vi "final_control_mk9_032425.vi"() -> ()   [LabVIEW 2023]
doc: "Simplified example program for initializing the COM port, determining the data frame of up to 26 Alicats, acquiring the data of the same number of Alicats, displaying the data of the one with the selected unit ID, and writing a setpoint to the same selected unit ID.\n\nThis is a slightly more feature rich version of the Alicat Simplified Driver Example, and contains an example of a method for interfacing with up to 26 Alicats on a single COM port by means of for loops with shift registers to handle sequential commands to each included Alicat. This also contains a method to write a setpoint to the same selected unit.\n\nIf coding for multiple Alicats on a single COM port without the use of for loops with shift registers, ensure that each Alicat command is executed sequentially. Alicat's RS-232/485 does not work if multiple devices are responding simultaneously."
uses:
  <vilib>/Platform/TimedLoop/XDataNode/timing_clust.ctl
  <vilib>/Platform/TimedLoop/XDataNode/nitl_modes.ctl
  <vilib>/Platform/TimedLoop/XDataNode/wakeup.ctl
  <vilib>/DAQmx/write.llb/DAQmx Write (Analog 1D DBL NChan 1Samp).vi
  <vilib>/DAQmx/read.llb/DAQmx Read (Analog DBL 1Chan 1Samp).vi
  <extravilib>/ChannelInstances/Tag-bool/Read With Abort.vi
  <extravilib>/ChannelInstances/Tag-bool/Write With Abort.vi
  <vilib>/Utility/file.llb/Write Delimited Spreadsheet (string).vi
  <extravilib>/ChannelInstances/Tag-bool/Instantiate.vi
  <vilib>/Utility/file.llb/Read Delimited Spreadsheet (DBL).vi
  <extravilib>/ChannelInstances/Tag-bool/EndpointRead.vi
  <vilib>/DAQmx/miscellaneous.llb/DAQmx Fill In Error Info.vi
  <extravilib>/ChannelInstances/Tag-bool/Endpoint.vi
  <vilib>/platform/TimedLoop/XDataNode/XDataNode.xnode
  <vilib>/express/express arith-compare/Formula/XNode/ExpressFormulaBlockNode.xnode
  <vilib>/Platform/TimedLoop/XDataNode/XDNodeRunTimeDep.lvlib
  <extravilib>/ChannelInstances/Tag-bool.lvlib
panel:
  in  "Tab Control":enum32{"Page 1", "Page 2"}(tab)
  in  "COM Port Settings":T1={"Baud Rate"=enum."19200", "VISA Sesssion In"="MassFlowControllers"}
  out "Range Exceeded":bool
  out "Error Present":bool
  out "Error Text":string
  out "Elapsed Time [ms]\n(all units)":dbl caption="Elapsed Time (s)"
  in  "Minimum time between \nreadings [ms] (all units)":u32
  in  "Device ID's \nto Include:":T2={"A"=TRUE, "B"=TRUE, "C"=TRUE, "D"=TRUE, "E"=TRUE, "F"=TRUE, "G"=FALSE, "H"=FALSE, "I"=FALSE, "J"=FALSE, "K"=FALSE, "L"=FALSE, "M"=FALSE, "N"=FALSE, "O"=FALSE, "P"=FALSE, "Q"=FALSE, "R"=FALSE, "S"=FALSE, "T"=FALSE, "U"=FALSE, "V"=FALSE, "W"=FALSE, "X"=FALSE, "Y"=FALSE, "Z"=FALSE}
  out "Active Device":u16(ring) items=["A", "B", "C", "D", "E", "F"]
  out "Meas. Data (for active device)":T3
  in  "Write File":path
  in  "Hold Time\n[min]":dbl=17.0 min=17.0
  out "N":i32
  in  "Read File":path
  in  "End Program":bool
  in  "Start From:":i32=1
  in  "t_read [ms]":dbl=24000.0
  out "T_SCh [C]":dbl format="%0.2f"
  out "iter start":string
  out "Iter_Duration [ms]":string
  out "C_SP [ppm]":string
  out "C_H2S [ppm]":string
  in  "Start Times":path
  out "len_SP":i32
  out "Setpoints":dbl[][](array[numeric])=[[4.2, 3.3], [69.0, 4.2]]
  out "Z":dbl[](array[numeric])
  out "ASP":dbl
  out "BSP":dbl
  out "CSP":dbl
  out "DSP":dbl
  out "ESP":dbl
  out "FSP":dbl
  out "N_read":i32
  out "Iter_#":string
  out "V_D":string
  out "V_H":string
  out "all rows":dbl[][](array[numeric])
  out "T_SCh":string
  out "Iteration Duration":i64
  out "read_cnt_true":i32
  out "iter_dur_read [ms]":i64
  out "t_diff":dbl
  out "date":string
  out "time":string
  # "Totalizer Timer"
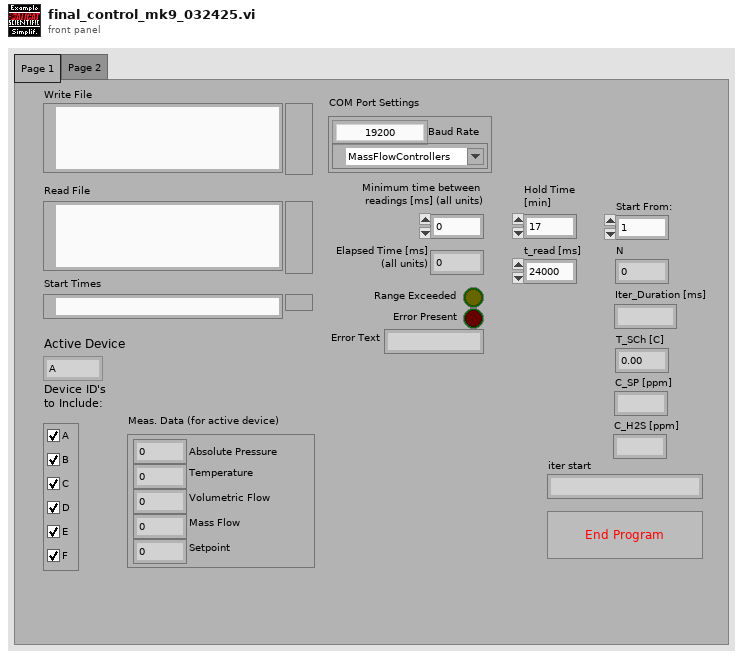
[diagram p1: front panel]
types:
  T1 = cluster{"Baud Rate":enum8{"2400", "9600", "19200", "38400", "57600", "115200", "Unknown"}, "VISA Sesssion In":refnum<visa-resource-name>}
  T2 = cluster{"A":bool, "B":bool, "C":bool, "D":bool, "E":bool, "F":bool, "G":bool, "H":bool, "I":bool, "J":bool, "K":bool, "L":bool, "M":bool, "N":bool, "O":bool, "P":bool, "Q":bool, "R":bool, "S":bool, "T":bool, "U":bool, "V":bool, "W":bool, "X":bool, "Y":bool, "Z":bool}
  T3 = cluster{"Absolute Pressure":dbl, "Gauge/Diff. Pressure":dbl, "Barometric Pressure":dbl, "Temperature":dbl, "Volumetric Flow":dbl, "Mass Flow":dbl, "Setpoint":dbl, "Valve Drive":dbl, "Totalizer":dbl, "[hr]":dbl, "[min]":dbl, "[sec]":dbl, "Totalizer Average Flow":dbl, "Totalizer Peak Flow":dbl, "Gas selected":string}
  T4 = cluster{"Unit ID":string, "Baud Rate":enum8{"2400", "9600", "19200", "38400", "57600", "115200", "Unknown"}, "VISA Sesssion In":refnum<visa-resource-name>}
  T5 = typedef "XDNodeRunTimeDep.lvlib/timing_clust.ctl" = cluster{"Expected End [f-1]":u64, "Actual End [f-1]":u64, "Finished Late? [f-1]":bool, "Expected End [i-1]":u64, "Actual End [i-1]":u64, "Finished Late? [i-1]":bool, "Expected Start [i]":u64, "Actual Start [i]":u64, "Expected Start [f]":u64, "Actual Start [f]":u64, "Source Name":string, "Structure Name":string, "Period":i64, "Deadline":i64, "Offset":i64, "Start":i64, "Priority":i32, "Timeout":i32, "Mode":T6, "Wakeup Reason":T7, "Error":errorcluster, "Source Type":string, "Secondary Source Type":string, "Global End Time":u64, "Global Start Time":u64, "Frame Duration":u64, "Iteration Duration":u64, "Assigned CPU":i32, "I/O Scan Engine Mode":u32}
  T6 = typedef "XDNodeRunTimeDep.lvlib/nitl_modes.ctl" = enum32{"No Change", "Process missed periods, maintain original phase", "Discard missed periods, maintain original phase", "Process missed periods, ignore original phase", "Discard missed periods, ignore original phase"}
  T7 = typedef "XDNodeRunTimeDep.lvlib/wakeup.ctl" = enum32{"Normal", "Aborted", "Asynchronous wakeup", "Timing source error", "Timed loop error", "Timeout"}
  T8 = typedef "Tag-bool.lvlib/))Channel.ctl" = refnum<queue>
  T9 = enum8{"2400", "9600", "19200", "38400", "57600", "115200", "Unknown"}
  T10 = cluster{"Absolute Pressure":bool, "Gauge/Diff. Pressure":bool, "Barometric Pressure":bool, "Temperature":bool, "Volumetric":bool, "Mass":bool, "Setpoint":bool, "Valve Drive":bool, "Totalizer":bool, "Totalizer Timer":bool, "Totalizer Average Flow":bool, "Totalizer Peak Flow":bool, "Gas Selected":bool, "Tot. Timer Format":u16}
  T11 = cluster{"Controller Full Scale":dbl, "Controller Select":u16, "Control Range":enum16{"Normal", "Inverted", "Bidirectional", "Unknown"}}
  T12 = cluster{"Controller Full Scale":dbl, "Controller Select":u16, "Control Range":enum16{"Normal", "Inverted", "Bidirectional", "Unknown"}}[]
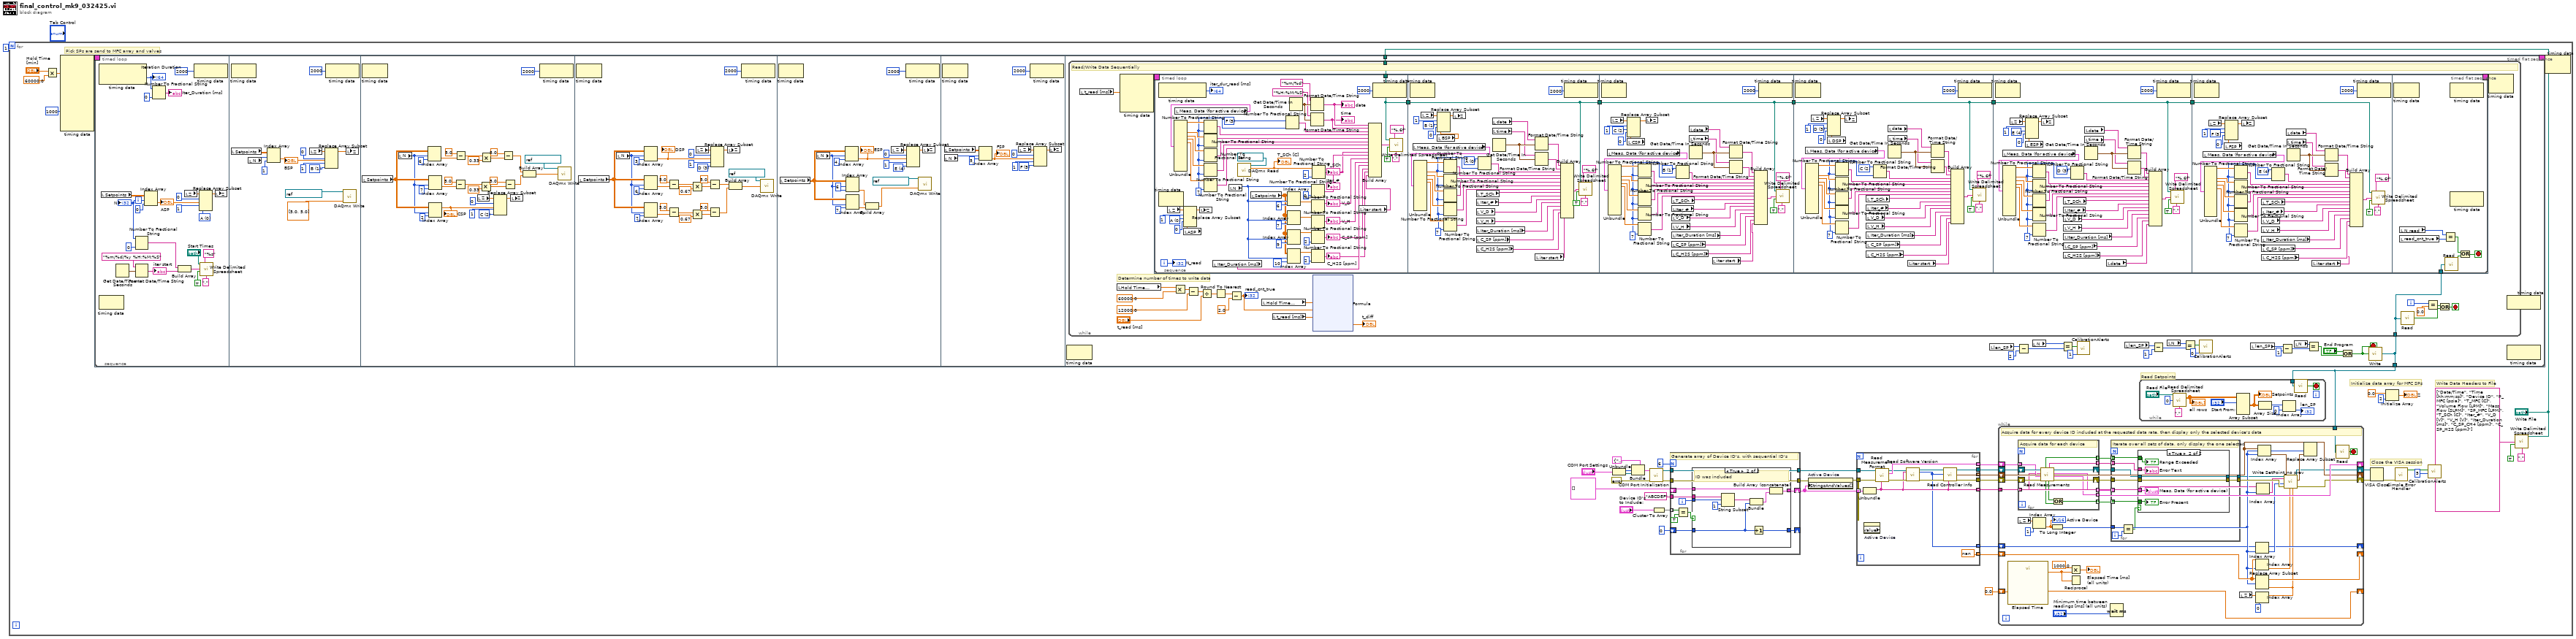
[diagram p0: block diagram]
diagram:
  n1 = for {
    N: 1 -> [_]
    # "Pick SPs are send to MFC array and valves"
    # "Write Data Headers to File"
    # "Read Setpoints"
    # "Initialize data array for MFC SPs"
    # "Close the VISA session"
    n2 = Multiply(x="Hold Time\n[min]", y=60000.0) -> (x*y=w5:dbl)
    n3 = node-c288(w5, i64 1000 ("Offset")) -> (w46:T5)  [unwired: 8 in]
    n4 = timed-loop "Write Data" {
      timing: w46 -> [_]
      timing-out: [_] -> w45
      tunnel: [w59] -> w12
      tunnel: "Write File" -> [w58]
      i -> [w67]
      stop <- w221 stop-if-true
      n5 = timed-sequence {
        timing: _ -> [_]
        timing-out: _ -> [_]
        tunnel: [w61] -> w59
        tunnel: w58 -> [w60]
        n6 = timed-flat-sequence {
          tunnel: [w216] -> w61
          tunnel: w60 -> [w217]
          frame #0 {
            w77 = u16 0 items=["A", "B", "C", "D", "E", "F"]
            n7 = node-c288() -> (w71:i64)  [unwired: 1 in, 1 out]
            "Iteration Duration" <- w71
            n8 = local read "Setpoints"() -> (w84:dbl[][])
            n9 = Get Date/Time In Seconds() -> (seconds since 1Jan1904=w72:timestamp)
            n10 = Number To Fractional String(number=w67, precision (6)=i16 0) -> (F-format string=w65:string)  [unwired: 2 in]
            n11 = Format Date/Time String(time format string (%c)="%m/%d/%y %H:%M:%S", seconds (now)=w72) -> (date/time string=w64:string)  [unwired: 1 in]
            "iter start" <- w64
            n12 = Index Array(array=w84, index (row)=w67, index (col)=0 ("index (row)")) -> (element=w82:dbl)
            "ASP" <- w82
            n13 = Number To Fractional String(number=w71, precision (6)=i16 0) -> (F-format string=→"Iter_Duration [ms]":string)  [unwired: 2 in]
            n14 = Build Array(w65, w64) -> (w63:string[])
            n15 = local read "Z"() -> (w80:dbl[])
            n16 = node-c288(i64 2000 ("Start")) -> ()  [unwired: 1 out]
            n17 = Replace Array Subset(array=w80, new element #1=w82, index #1=0 ("index"), new element #2=w77, index #2=1 ("index")) -> (w81:dbl[])
            n18 = call-poly <vilib>:"Write Delimited Spreadsheet.vi"("file path (dialog if empty)"="Start Times", "format (%s)"="%s" ("format (%.3f)"), "1D data"=w63, "append to file? (new file:F)"=TRUE, "delimiter (\\t)"="," ("delimiter (\\t)")) -> ()  [unwired: 9 in, 2 out]
            n19 = local write "Z"(w81) -> ()
            "N" <- w67
          }
          frame #1 {
            w92 = u16 1 items=["A", "B", "C", "D", "E", "F"]
            n20 = node-c288() -> ()  [unwired: 1 in, 1 out]
            n21 = local read "Setpoints"() -> (w100:dbl[][])
            n22 = local read "N"() -> (w93:i32)
            n23 = Index Array(array=w100, index (row)=w93, index (col)=1 ("index (row)")) -> (element=w97:dbl)
            "BSP" <- w97
            n24 = local read "Z"() -> (w95:dbl[])
            n25 = Replace Array Subset(array=w95, new element #1=w97, index #1=0 ("index"), new element #2=w92, index #2=1 ("index")) -> (w96:dbl[])
            n26 = node-c288(i64 2000 ("Start")) -> ()  [unwired: 1 out]
            n27 = call-poly <vilib>:"DAQmx Write.vi"("task/channels in"=refnum<k21> "Valve_cont", "data"=dbl[] [5.0, 5.0]) -> ()  [unwired: 11 in, 3 out]
            n28 = local write "Z"(w96) -> ()
          }
          frame #2 {
            w107 = u16 2 items=["A", "B", "C", "D", "E", "F"]
            n29 = node-c288() -> ()  [unwired: 1 in, 1 out]
            n30 = local read "Setpoints"() -> (w119:dbl[][])
            n31 = local read "N"() -> (w118:i32)
            n32 = Index Array(array=w119, index (row)=w118, index (col)=6 ("disabled index (col)")) -> (element=w109:dbl)
            n33 = Index Array(array=w119, index (row)=w118, index (col)=7 ("disabled index (col)")) -> (element=w117:dbl)
            n34 = Index Array(array=w119, index (row)=w118, index (col)=2 ("index (row)")) -> (element=w131:dbl)
            "CSP" <- w131
            n35 = Subtract(x=5.0, y=w117) -> (x-y=w126:dbl)
            n36 = Subtract(x=5.0, y=w109) -> (x-y=w113:dbl)
            n37 = local read "Z"() -> (w129:dbl[])
            n38 = Multiply(x=w126, y=0.33) -> (x*y=w124:dbl)
            n39 = Multiply(x=w113, y=0.33) -> (x*y=w111:dbl)
            n40 = Replace Array Subset(array=w129, new element #1=w131, index #1=0 ("index"), new element #2=w107, index #2=1 ("index")) -> (w130:dbl[])
            n41 = Subtract(x=5.0, y=w111) -> (x-y=w108:dbl)
            n42 = Subtract(x=5.0, y=w124) -> (x-y=w121:dbl)
            n43 = local write "Z"(w130) -> ()
            n44 = Build Array(w108, w121) -> (w120:dbl[])
            n45 = node-c288(i64 2000 ("Start")) -> ()  [unwired: 1 out]
            n46 = call-poly <vilib>:"DAQmx Write.vi"("task/channels in"=refnum<k21> "Valve_cont", "data"=w120) -> ()  [unwired: 11 in, 3 out]
          }
          frame #3 {
            w158 = u16 3 items=["A", "B", "C", "D", "E", "F"]
            n47 = node-c288() -> ()  [unwired: 1 in, 1 out]
            n48 = local read "Setpoints"() -> (w147:dbl[][])
            n49 = local read "N"() -> (w146:i32)
            n50 = Index Array(array=w147, index (row)=w146, index (col)=7 ("disabled index (col)")) -> (element=w139:dbl)
            n51 = Index Array(array=w147, index (row)=w146, index (col)=3 ("index (row)")) -> (element=w162:dbl)
            "DSP" <- w162
            n52 = Index Array(array=w147, index (row)=w146, index (col)=6 ("disabled index (col)")) -> (element=w145:dbl)
            n53 = Subtract(x=5.0, y=w145) -> (x-y=w155:dbl)
            n54 = Subtract(x=5.0, y=w139) -> (x-y=w143:dbl)
            n55 = Multiply(x=w155, y=0.67) -> (x*y=w153:dbl)
            n56 = Multiply(x=w143, y=0.67) -> (x*y=w141:dbl)
            n57 = local read "Z"() -> (w160:dbl[])
            n58 = Subtract(x=5.0, y=w153) -> (x-y=w149:dbl)
            n59 = Subtract(x=5.0, y=w141) -> (x-y=w138:dbl)
            n60 = Replace Array Subset(array=w160, new element #1=w162, index #1=0 ("index"), new element #2=w158, index #2=1 ("index")) -> (w161:dbl[])
            n61 = local write "Z"(w161) -> ()
            n62 = Build Array(w149, w138) -> (w148:dbl[])
            n63 = node-c288(i64 2000 ("Start")) -> ()  [unwired: 1 out]
            n64 = call-poly <vilib>:"DAQmx Write.vi"("task/channels in"=refnum<k21> "Valve_cont", "data"=w148) -> ()  [unwired: 11 in, 3 out]
          }
          frame #4 {
            w179 = u16 4 items=["A", "B", "C", "D", "E", "F"]
            n65 = node-c288() -> ()  [unwired: 1 in, 1 out]
            n66 = local read "Setpoints"() -> (w174:dbl[][])
            n67 = local read "N"() -> (w173:i32)
            n68 = Index Array(array=w174, index (row)=w173, index (col)=4 ("index (row)")) -> (element=w183:dbl)
            "ESP" <- w183
            n69 = Index Array(array=w174, index (row)=w173, index (col)=6 ("disabled index (col)")) -> (element=w176:dbl)
            n70 = Index Array(array=w174, index (row)=w173, index (col)=7 ("disabled index (col)")) -> (element=w175:dbl)
            n71 = Build Array(w176, w175) -> (w172:dbl[])
            n72 = local read "Z"() -> (w181:dbl[])
            n73 = node-c288(i64 2000 ("Start")) -> ()  [unwired: 1 out]
            n74 = Replace Array Subset(array=w181, new element #1=w183, index #1=0 ("index"), new element #2=w179, index #2=1 ("index")) -> (w182:dbl[])
            n75 = call-poly <vilib>:"DAQmx Write.vi"("task/channels in"=refnum<k21> "Valve_cont", "data"=w172) -> ()  [unwired: 11 in, 3 out]
            n76 = local write "Z"(w182) -> ()
          }
          frame #5 {
            w193 = u16 5 items=["A", "B", "C", "D", "E", "F"]
            n77 = node-c288() -> ()  [unwired: 1 in, 1 out]
            n78 = local read "Setpoints"() -> (w196:dbl[][])
            n79 = local read "N"() -> (w191:i32)
            n80 = Index Array(array=w196, index (row)=w191, index (col)=5 ("index (row)")) -> (element=w192:dbl)
            "FSP" <- w192
            n81 = local read "Z"() -> (w195:dbl[])
            n82 = node-c288(i64 2000 ("Start")) -> ()  [unwired: 1 out]
            n83 = Replace Array Subset(array=w195, new element #1=w192, index #1=0 ("index"), new element #2=w193, index #2=1 ("index")) -> (w194:dbl[])
            n84 = local write "Z"(w194) -> ()
          }
          frame #6 {
            n85 = node-c288() -> ()  [unwired: 1 in, 1 out]
            n86 = local read "len_SP"() -> (w207:i32)
            n87 = Subtract(x=w207, y=2) -> (x-y=w209:i32)
            n88 = local read "N"() -> (w208:i32)
            n89 = Equal?(x=w208, y=w209) -> (x = y?=w205:bool)
            n90 = call "CalibrationAlerts.vi"("Alert Type (0)"=1, "Trigger"=w205) -> ()  [unwired: 10 in]
            n91 = local read "len_SP"() -> (w212:i32)
            n92 = Subtract(x=w212, y=1) -> (x-y=w211:i32)
            n93 = local read "N"() -> (w215:i32)
            n94 = Equal?(x=w215, y=w211) -> (x = y?=w204:bool)
            n95 = call "CalibrationAlerts.vi"("Alert Type (0)"=0, "Trigger"=w204) -> ()  [unwired: 10 in]
            n96 = local read "len_SP"() -> (w220:i32)
            n97 = Subtract(x=w220, y=1) -> (x-y=w223:i32)
            n98 = local read "N"() -> (w219:i32)
            n99 = Equal?(x=w219, y=w223) -> (x = y?=w222:bool)
            n100 = Or(x="End Program", y=w222) -> (x .or. y?=w221:bool)
            n101 = call <extravilib>:"Write.vi"("element"=w221) -> ("channel"=w216:T8)  [unwired: 1 out]
            n102 = while {
              tunnel: w217 -> [w245]
              tunnel: w216 -> [w235]
              i -> [w234]
              stop <- w241 stop-if-true
              # "Determine number of times to write data"
              # "Read/Write Data Sequentially"
              n103 = local read "t_read [ms]"() -> (w225:dbl)
              n104 = local read "Hold Time\n[min]"() -> (w239:dbl)
              n105 = node-c288(w225) -> (w247:T5)  [unwired: 3 in]
              n106 = timed-loop {
                timing: w247 -> [_]
                timing-out: [_] -> w246
                tunnel: w245 -> [w260]
                tunnel: w235 -> [w261]
                i -> [w325]
                stop <- w549 stop-if-true
                n107 = timed-sequence {
                  timing: _ -> [_]
                  timing-out: _ -> [_]
                  tunnel: w261 -> [w263]
                  tunnel: w260 -> [w262]
                  n108 = timed-flat-sequence {
                    tunnel: [w291] -> w268
                    tunnel: w262 -> [w291]
                    tunnel: w268 -> [w357]
                    tunnel: [w357] -> w267
                    tunnel: w267 -> [w393]
                    tunnel: [w393] -> w266
                    tunnel: w266 -> [w432]
                    tunnel: [w432] -> w265
                    tunnel: w265 -> [w465]
                    tunnel: [w465] -> w264
                    tunnel: w264 -> [w518]
                    tunnel: w263 -> [w548]
                    frame #0 {
                      w306 = u16 5 items=["A", "B", "C", "D", "E", "F"]
                      w309 = u16 0 items=["A", "B", "C", "D", "E", "F"]
                      w302 = i16 7 ("precision (6)")
                      n109 = node-c288() -> (→"iter_dur_read [ms]":i64)  [unwired: 1 in]
                      n110 = local read "Z"() -> (w295:dbl[])
                      n111 = local read "Meas. Data (for active device)"() -> (w292:T3)
                      n112 = Unbundle(w292) -> ("Absolute Pressure"=w315:dbl, "Temperature"=w305:dbl, "Volumetric Flow"=w311:dbl, "Mass Flow"=w304:dbl, "Setpoint"=w303:dbl)  [unwired: 10 out]
                      n113 = local read "ASP"() -> (w293:dbl)
                      n114 = Replace Array Subset(array=w295, new element #1=w309, index #1=1 ("index"), new element #2=w293, index #2=0 ("index")) -> (w294:dbl[])
                      n115 = local write "Z"(w294) -> ()
                      n116 = Number To Fractional String(number=w315, precision (6)=w302) -> (F-format string=w300:string)  [unwired: 2 in]
                      n117 = Number To Fractional String(number=w305, precision (6)=w302) -> (F-format string=w298:string)  [unwired: 2 in]
                      n118 = Number To Fractional String(number=w311, precision (6)=w302) -> (F-format string=w299:string)  [unwired: 2 in]
                      n119 = Number To Fractional String(number=w304, precision (6)=w302) -> (F-format string=w297:string)  [unwired: 2 in]
                      n120 = Number To Fractional String(number=w303, precision (6)=w302) -> (F-format string=w296:string)  [unwired: 2 in]
                      n121 = local read "Iter_Duration [ms]"() -> (w290:string)
                      n122 = local read "N"() -> (w272:i32)
                      n123 = call-poly <vilib>:"DAQmx Read.vi"("task/channels in"=refnum<k21> "T_SCh") -> ("data"=w318:dbl)  [unwired: 12 in, 2 out]
                      "T_SCh [C]" <- w318
                      n124 = local read "Setpoints"() -> (w271:dbl[][])
                      n125 = Number To Fractional String(number=w306, precision (6)=w302) -> (F-format string=w301:string)  [unwired: 2 in]
                      n126 = Index Array(array=w271, index (row)=w272, index (col)=6 ("disabled index (col)")) -> (element=w322:dbl)
                      n127 = Index Array(array=w271, index (row)=w272, index (col)=7 ("disabled index (col)")) -> (element=w321:dbl)
                      n128 = Index Array(array=w271, index (row)=w272, index (col)=9 ("disabled index (col)")) -> (element=w278:dbl)
                      n129 = Index Array(array=w271, index (row)=w272, index (col)=10 ("disabled index (col)")) -> (element=w274:dbl)
                      n130 = Get Date/Time In Seconds() -> (seconds since 1Jan1904=w284:timestamp)
                      n131 = Format Date/Time String(time format string (%c)="%m/%d", seconds (now)=w284) -> (date/time string=w286:string)  [unwired: 1 in]
                      "date" <- w286
                      n132 = Format Date/Time String(time format string (%c)="%H:%M:%S", seconds (now)=w284) -> (date/time string=w285:string)  [unwired: 1 in]
                      "time" <- w285
                      n133 = Number To Fractional String(number=w272, precision (6)=i16 0) -> (F-format string=w287:string)  [unwired: 2 in]
                      "Iter_#" <- w287
                      n134 = Number To Fractional String(number=w322) -> (F-format string=w288:string)  [unwired: 3 in]
                      "V_D" <- w288
                      n135 = Number To Fractional String(number=w321) -> (F-format string=w289:string)  [unwired: 3 in]
                      "V_H" <- w289
                      n136 = Number To Fractional String(number=w278, precision (6)=i16 2) -> (F-format string=w276:string)  [unwired: 2 in]
                      "C_SP [ppm]" <- w276
                      n137 = Number To Fractional String(number=w274, precision (6)=i16 2) -> (F-format string=w270:string)  [unwired: 2 in]
                      "C_H2S [ppm]" <- w270
                      n138 = Number To Fractional String(number=w318, precision (6)=i16 2) -> (F-format string=w281:string)  [unwired: 2 in]
                      "T_SCh" <- w281
                      n139 = local read "iter start"() -> (w269:string)
                      n140 = Build Array(w286, w285, w301, w300, w298, w299, w297, w296, w281, w287, w288, w289, w290, w276, w270, w269) -> (w312:string[])
                      n141 = node-c288(i64 2000 ("Start")) -> ()  [unwired: 1 out]
                      n142 = call-poly <vilib>:"Write Delimited Spreadsheet.vi"("file path (dialog if empty)"=w291, "format (%s)"="%.6f" ("format (%.3f)"), "1D data"=w312, "append to file? (new file:F)"=TRUE, "delimiter (\\t)"="," ("delimiter (\\t)")) -> ()  [unwired: 9 in, 2 out]
                      "N_read" <- w325
                    }
                    frame #1 {
                      w354 = u16 0 items=["A", "B", "C", "D", "E", "F"]
                      w363 = u16 1 items=["A", "B", "C", "D", "E", "F"]
                      w350 = i16 7 ("precision (6)")
                      n143 = node-c288() -> ()  [unwired: 1 in, 1 out]
                      n144 = local read "Meas. Data (for active device)"() -> (w361:T3)
                      n145 = Unbundle(w361) -> ("Absolute Pressure"=w369:dbl, "Temperature"=w353:dbl, "Volumetric Flow"=w365:dbl, "Mass Flow"=w352:dbl, "Setpoint"=w351:dbl)  [unwired: 10 out]
                      n146 = local read "Z"() -> (w360:dbl[])
                      n147 = local read "BSP"() -> (w355:dbl)
                      n148 = Replace Array Subset(array=w360, new element #1=w363, index #1=1 ("index"), new element #2=w355, index #2=0 ("index")) -> (w359:dbl[])
                      n149 = Number To Fractional String(number=w369, precision (6)=w350) -> (F-format string=w348:string)  [unwired: 2 in]
                      n150 = Number To Fractional String(number=w353, precision (6)=w350) -> (F-format string=w346:string)  [unwired: 2 in]
                      n151 = Number To Fractional String(number=w365, precision (6)=w350) -> (F-format string=w347:string)  [unwired: 2 in]
                      n152 = Number To Fractional String(number=w352, precision (6)=w350) -> (F-format string=w345:string)  [unwired: 2 in]
                      n153 = Number To Fractional String(number=w351, precision (6)=w350) -> (F-format string=w344:string)  [unwired: 2 in]
                      n154 = local write "Z"(w359) -> ()
                      n155 = local read "T_SCh"() -> (w343:string)
                      n156 = local read "Iter_#"() -> (w342:string)
                      n157 = local read "V_D"() -> (w341:string)
                      n158 = local read "V_H"() -> (w340:string)
                      n159 = local read "Iter_Duration [ms]"() -> (w339:string)
                      n160 = local read "C_SP [ppm]"() -> (w333:string)
                      n161 = local read "C_H2S [ppm]"() -> (w332:string)
                      n162 = Number To Fractional String(number=w354, precision (6)=w350) -> (F-format string=w349:string)  [unwired: 2 in]
                      n163 = local read "date"() -> (w334:string)
                      n164 = local read "time"() -> (w335:string)
                      n165 = Get Date/Time In Seconds() -> (seconds since 1Jan1904=w336:timestamp)
                      n166 = Format Date/Time String(time format string (%c)=w334, seconds (now)=w336) -> (date/time string=w338:string)  [unwired: 1 in]
                      n167 = Format Date/Time String(time format string (%c)=w335, seconds (now)=w336) -> (date/time string=w337:string)  [unwired: 1 in]
                      n168 = local read "iter start"() -> (w331:string)
                      n169 = Build Array(w338, w337, w349, w348, w346, w347, w345, w344, w343, w342, w341, w340, w339, w333, w332, w331) -> (w366:string[])
                      n170 = node-c288(i64 2000 ("Start")) -> ()  [unwired: 1 out]
                      n171 = call-poly <vilib>:"Write Delimited Spreadsheet.vi"("file path (dialog if empty)"=w357, "format (%s)"="%.6f" ("format (%.3f)"), "1D data"=w366, "append to file? (new file:F)"=TRUE, "delimiter (\\t)"="," ("delimiter (\\t)")) -> ()  [unwired: 9 in, 2 out]
                    }
                    frame #2 {
                      w399 = u16 1 items=["A", "B", "C", "D", "E", "F"]
                      w398 = i16 7 ("precision (6)")
                      w411 = u16 2 items=["A", "B", "C", "D", "E", "F"]
                      n172 = node-c288() -> ()  [unwired: 1 in, 1 out]
                      n173 = local read "Meas. Data (for active device)"() -> (w400:T3)
                      n174 = Unbundle(w400) -> ("Absolute Pressure"=w405:dbl, "Temperature"=w403:dbl, "Volumetric Flow"=w404:dbl, "Mass Flow"=w402:dbl, "Setpoint"=w401:dbl)  [unwired: 10 out]
                      n175 = local read "Z"() -> (w410:dbl[])
                      n176 = local read "CSP"() -> (w406:dbl)
                      n177 = Replace Array Subset(array=w410, new element #1=w411, index #1=1 ("index"), new element #2=w406, index #2=0 ("index")) -> (w409:dbl[])
                      n178 = Number To Fractional String(number=w405, precision (6)=w398) -> (F-format string=w386:string)  [unwired: 2 in]
                      n179 = Number To Fractional String(number=w403, precision (6)=w398) -> (F-format string=w385:string)  [unwired: 2 in]
                      n180 = Number To Fractional String(number=w404, precision (6)=w398) -> (F-format string=w384:string)  [unwired: 2 in]
                      n181 = Number To Fractional String(number=w402, precision (6)=w398) -> (F-format string=w383:string)  [unwired: 2 in]
                      n182 = Number To Fractional String(number=w401, precision (6)=w398) -> (F-format string=w382:string)  [unwired: 2 in]
                      n183 = local write "Z"(w409) -> ()
                      n184 = local read "T_SCh"() -> (w392:string)
                      n185 = local read "Iter_#"() -> (w391:string)
                      n186 = local read "V_D"() -> (w390:string)
                      n187 = local read "V_H"() -> (w389:string)
                      n188 = local read "Iter_Duration [ms]"() -> (w388:string)
                      n189 = local read "C_SP [ppm]"() -> (w376:string)
                      n190 = local read "C_H2S [ppm]"() -> (w375:string)
                      n191 = Number To Fractional String(number=w399, precision (6)=w398) -> (F-format string=w387:string)  [unwired: 2 in]
                      n192 = local read "date"() -> (w377:string)
                      n193 = local read "time"() -> (w378:string)
                      n194 = Get Date/Time In Seconds() -> (seconds since 1Jan1904=w379:timestamp)
                      n195 = local read "iter start"() -> (w374:string)
                      n196 = Format Date/Time String(time format string (%c)=w377, seconds (now)=w379) -> (date/time string=w381:string)  [unwired: 1 in]
                      n197 = Format Date/Time String(time format string (%c)=w378, seconds (now)=w379) -> (date/time string=w380:string)  [unwired: 1 in]
                      n198 = Build Array(w381, w380, w387, w386, w385, w384, w383, w382, w392, w391, w390, w389, w388, w376, w375, w374) -> (w394:string[])
                      n199 = node-c288(i64 2000 ("Start")) -> ()  [unwired: 1 out]
                      n200 = call-poly <vilib>:"Write Delimited Spreadsheet.vi"("file path (dialog if empty)"=w393, "format (%s)"="%.6f" ("format (%.3f)"), "1D data"=w394, "append to file? (new file:F)"=TRUE, "delimiter (\\t)"="," ("delimiter (\\t)")) -> ()  [unwired: 9 in, 2 out]
                    }
                    frame #3 {
                      w426 = u16 3 items=["A", "B", "C", "D", "E", "F"]
                      w449 = u16 2 items=["A", "B", "C", "D", "E", "F"]
                      w448 = i16 7 ("precision (6)")
                      n201 = node-c288() -> ()  [unwired: 1 in, 1 out]
                      n202 = local read "Meas. Data (for active device)"() -> (w431:T3)
                      n203 = Unbundle(w431) -> ("Absolute Pressure"=w454:dbl, "Temperature"=w452:dbl, "Volumetric Flow"=w453:dbl, "Mass Flow"=w451:dbl, "Setpoint"=w450:dbl)  [unwired: 10 out]
                      n204 = local read "Z"() -> (w429:dbl[])
                      n205 = local read "DSP"() -> (w430:dbl)
                      n206 = Replace Array Subset(array=w429, new element #1=w426, index #1=1 ("index"), new element #2=w430, index #2=0 ("index")) -> (w428:dbl[])
                      n207 = Number To Fractional String(number=w454, precision (6)=w448) -> (F-format string=w442:string)  [unwired: 2 in]
                      n208 = Number To Fractional String(number=w452, precision (6)=w448) -> (F-format string=w441:string)  [unwired: 2 in]
                      n209 = Number To Fractional String(number=w453, precision (6)=w448) -> (F-format string=w440:string)  [unwired: 2 in]
                      n210 = Number To Fractional String(number=w451, precision (6)=w448) -> (F-format string=w439:string)  [unwired: 2 in]
                      n211 = Number To Fractional String(number=w450, precision (6)=w448) -> (F-format string=w438:string)  [unwired: 2 in]
                      n212 = local write "Z"(w428) -> ()
                      n213 = local read "T_SCh"() -> (w433:string)
                      n214 = local read "Iter_#"() -> (w434:string)
                      n215 = local read "V_D"() -> (w435:string)
                      n216 = local read "V_H"() -> (w436:string)
                      n217 = local read "Iter_Duration [ms]"() -> (w437:string)
                      n218 = local read "C_SP [ppm]"() -> (w419:string)
                      n219 = local read "C_H2S [ppm]"() -> (w418:string)
                      n220 = Number To Fractional String(number=w449, precision (6)=w448) -> (F-format string=w443:string)  [unwired: 2 in]
                      n221 = local read "date"() -> (w420:string)
                      n222 = local read "time"() -> (w421:string)
                      n223 = Get Date/Time In Seconds() -> (seconds since 1Jan1904=w422:timestamp)
                      n224 = local read "iter start"() -> (w417:string)
                      n225 = Format Date/Time String(time format string (%c)=w420, seconds (now)=w422) -> (date/time string=w424:string)  [unwired: 1 in]
                      n226 = Format Date/Time String(time format string (%c)=w421, seconds (now)=w422) -> (date/time string=w423:string)  [unwired: 1 in]
                      n227 = Build Array(w424, w423, w443, w442, w441, w440, w439, w438, w433, w434, w435, w436, w437, w419, w418, w417) -> (w444:string[])
                      n228 = node-c288(i64 2000 ("Start")) -> ()  [unwired: 1 out]
                      n229 = call-poly <vilib>:"Write Delimited Spreadsheet.vi"("file path (dialog if empty)"=w432, "format (%s)"="%.6f" ("format (%.3f)"), "1D data"=w444, "append to file? (new file:F)"=TRUE, "delimiter (\\t)"="," ("delimiter (\\t)")) -> ()  [unwired: 9 in, 2 out]
                    }
                    frame #4 {
                      w473 = u16 4 items=["A", "B", "C", "D", "E", "F"]
                      w492 = u16 3 items=["A", "B", "C", "D", "E", "F"]
                      w491 = i16 7 ("precision (6)")
                      n230 = node-c288() -> ()  [unwired: 1 in, 1 out]
                      n231 = local read "Meas. Data (for active device)"() -> (w475:T3)
                      n232 = Unbundle(w475) -> ("Absolute Pressure"=w497:dbl, "Temperature"=w495:dbl, "Volumetric Flow"=w496:dbl, "Mass Flow"=w494:dbl, "Setpoint"=w493:dbl)  [unwired: 10 out]
                      n233 = local read "Z"() -> (w470:dbl[])
                      n234 = local read "ESP"() -> (w471:dbl)
                      n235 = Replace Array Subset(array=w470, new element #1=w473, index #1=1 ("index"), new element #2=w471, index #2=0 ("index")) -> (w469:dbl[])
                      n236 = Number To Fractional String(number=w497, precision (6)=w491) -> (F-format string=w485:string)  [unwired: 2 in]
                      n237 = Number To Fractional String(number=w495, precision (6)=w491) -> (F-format string=w484:string)  [unwired: 2 in]
                      n238 = Number To Fractional String(number=w496, precision (6)=w491) -> (F-format string=w483:string)  [unwired: 2 in]
                      n239 = Number To Fractional String(number=w494, precision (6)=w491) -> (F-format string=w482:string)  [unwired: 2 in]
                      n240 = Number To Fractional String(number=w493, precision (6)=w491) -> (F-format string=w481:string)  [unwired: 2 in]
                      n241 = local write "Z"(w469) -> ()
                      n242 = local read "T_SCh"() -> (w480:string)
                      n243 = local read "Iter_#"() -> (w476:string)
                      n244 = local read "V_D"() -> (w477:string)
                      n245 = local read "V_H"() -> (w478:string)
                      n246 = local read "Iter_Duration [ms]"() -> (w479:string)
                      n247 = local read "C_SP [ppm]"() -> (w462:string)
                      n248 = local read "C_H2S [ppm]"() -> (w461:string)
                      n249 = Number To Fractional String(number=w492, precision (6)=w491) -> (F-format string=w486:string)  [unwired: 2 in]
                      n250 = local read "date"() -> (w463:string)
                      n251 = local read "time"() -> (w464:string)
                      n252 = Get Date/Time In Seconds() -> (seconds since 1Jan1904=w466:timestamp)
                      n253 = local read "date"() -> (w460:string)
                      n254 = Format Date/Time String(time format string (%c)=w463, seconds (now)=w466) -> (date/time string=w468:string)  [unwired: 1 in]
                      n255 = Format Date/Time String(time format string (%c)=w464, seconds (now)=w466) -> (date/time string=w467:string)  [unwired: 1 in]
                      n256 = Build Array(w468, w467, w486, w485, w484, w483, w482, w481, w480, w476, w477, w478, w479, w462, w461, w460) -> (w487:string[])
                      n257 = node-c288(i64 2000 ("Start")) -> ()  [unwired: 1 out]
                      n258 = call-poly <vilib>:"Write Delimited Spreadsheet.vi"("file path (dialog if empty)"=w465, "format (%s)"="%.6f" ("format (%.3f)"), "1D data"=w487, "append to file? (new file:F)"=TRUE, "delimiter (\\t)"="," ("delimiter (\\t)")) -> ()  [unwired: 9 in, 2 out]
                    }
                    frame #5 {
                      w516 = u16 5 items=["A", "B", "C", "D", "E", "F"]
                      w536 = u16 4 items=["A", "B", "C", "D", "E", "F"]
                      w535 = i16 7 ("precision (6)")
                      n259 = node-c288() -> ()  [unwired: 1 in, 1 out]
                      n260 = local read "Meas. Data (for active device)"() -> (w519:T3)
                      n261 = Unbundle(w519) -> ("Absolute Pressure"=w541:dbl, "Temperature"=w539:dbl, "Volumetric Flow"=w540:dbl, "Mass Flow"=w538:dbl, "Setpoint"=w537:dbl)  [unwired: 10 out]
                      n262 = local read "Z"() -> (w512:dbl[])
                      n263 = local read "FSP"() -> (w514:dbl)
                      n264 = Replace Array Subset(array=w512, new element #1=w516, index #1=1 ("index"), new element #2=w514, index #2=0 ("index")) -> (w513:dbl[])
                      n265 = Number To Fractional String(number=w541, precision (6)=w535) -> (F-format string=w529:string)  [unwired: 2 in]
                      n266 = Number To Fractional String(number=w539, precision (6)=w535) -> (F-format string=w528:string)  [unwired: 2 in]
                      n267 = Number To Fractional String(number=w540, precision (6)=w535) -> (F-format string=w527:string)  [unwired: 2 in]
                      n268 = Number To Fractional String(number=w538, precision (6)=w535) -> (F-format string=w526:string)  [unwired: 2 in]
                      n269 = Number To Fractional String(number=w537, precision (6)=w535) -> (F-format string=w525:string)  [unwired: 2 in]
                      n270 = local write "Z"(w513) -> ()
                      n271 = local read "T_SCh"() -> (w520:string)
                      n272 = local read "Iter_#"() -> (w521:string)
                      n273 = local read "V_D"() -> (w522:string)
                      n274 = local read "V_H"() -> (w523:string)
                      n275 = local read "Iter_Duration [ms]"() -> (w524:string)
                      n276 = local read "C_SP [ppm]"() -> (w506:string)
                      n277 = local read "C_H2S [ppm]"() -> (w505:string)
                      n278 = Number To Fractional String(number=w536, precision (6)=w535) -> (F-format string=w530:string)  [unwired: 2 in]
                      n279 = local read "date"() -> (w507:string)
                      n280 = local read "time"() -> (w508:string)
                      n281 = Get Date/Time In Seconds() -> (seconds since 1Jan1904=w509:timestamp)
                      n282 = local read "iter start"() -> (w504:string)
                      n283 = Format Date/Time String(time format string (%c)=w507, seconds (now)=w509) -> (date/time string=w511:string)  [unwired: 1 in]
                      n284 = Format Date/Time String(time format string (%c)=w508, seconds (now)=w509) -> (date/time string=w510:string)  [unwired: 1 in]
                      n285 = Build Array(w511, w510, w530, w529, w528, w527, w526, w525, w520, w521, w522, w523, w524, w506, w505, w504) -> (w531:string[])
                      n286 = node-c288(i64 2000 ("Start")) -> ()  [unwired: 1 out]
                      n287 = call-poly <vilib>:"Write Delimited Spreadsheet.vi"("file path (dialog if empty)"=w518, "format (%s)"="%.6f" ("format (%.3f)"), "1D data"=w531, "append to file? (new file:F)"=TRUE, "delimiter (\\t)"="," ("delimiter (\\t)")) -> ()  [unwired: 9 in, 2 out]
                    }
                    frame #6 {
                      n288 = node-c288() -> ()  [unwired: 1 in, 1 out]
                      n289 = local read "N_read"() -> (w546:i32)
                      n290 = local read "read_cnt_true"() -> (w547:i32)
                      n291 = Equal?(x=w546, y=w547) -> (x = y?=w551:bool)
                      n292 = call <extravilib>:"Read.vi"("channel"=w548) -> ("element"=w550:bool)  [unwired: 1 in, 1 out]
                      n293 = node-c288() -> ()  [unwired: 1 in, 1 out]
                      n294 = Or(x=w551, y=w550) -> (x .or. y?=w549:bool)
                    }
                  }
                }
                n295 = node-c288() -> ()  [unwired: 1 in, 1 out]
                n296 = node-c288() -> ()  [unwired: 1 in, 1 out]
              }
              n297 = Multiply(x=w239, y=60000.0) -> (x*y=w238:dbl)
              n298 = Subtract(x=w238, y=12000.0) -> (x-y=w236:dbl)
              n299 = Divide(x=w236, y="t_read [ms]") -> (x/y=w232:dbl)
              n300 = Round To Nearest(number=w232) -> (nearest integer value=w231:dbl)
              n301 = Subtract(x=w231, y=2.0) -> (x-y=w226:dbl)
              "read_cnt_true" <- w226
              n302 = local read "Hold Time\n[min]"() -> (w228:dbl)
              n303 = local read "t_read [ms]"() -> (w227:dbl)
              n304 = xnode "Formula"("X1"=w228, "X2"=w226, "X3"=w227) -> ("Result"=→"t_diff":dbl)  [unwired: 1 in, 1 out]
              n305 = call <extravilib>:"Read.vi"("channel"=w235) -> ("element"=w242:bool)  [unwired: 1 in, 1 out]
              n306 = Equal?(x=w234, y=0.0) -> (x = y?=w243:bool)
              n307 = Or(x=w243, y=w242) -> (x .or. y?=w241:bool)
              n308 = node-c288(w246) -> ()  [unwired: 1 out]
            }
            n309 = node-c288() -> ()  [unwired: 1 in, 1 out]
          }
        }
      }
      n310 = node-c288() -> ()  [unwired: 1 in, 1 out]
      n311 = node-c288() -> ()  [unwired: 1 in, 1 out]
    }
    n312 = Unbundle("COM Port Settings") -> ("Baud Rate"=w37:T9, "VISA Sesssion In"=w36:refnum<visa-resource-name>)
    n313 = Bundle(cluster=T4 {"Unit ID"="A", "Baud Rate"=enum."19200", "VISA Sesssion In"="COM1"} ("Communication Settings"), "Baud Rate"=w37, "VISA Sesssion In"=w36) -> (w35:T4)  [unwired: 1 in]
    n314 = call "COM Port Initialization.vi"("error in (no error)"=errorcluster {"status"=FALSE, "code"=0, "source"=""}, "Communication Settings"=w35) -> ("error out"=w28:errorcluster, "VISA Session Out"=w27:refnum<visa-resource-name>)  [unwired: 8 in]
    n315 = Cluster To Array(cluster="Device ID's \nto Include:") -> (array=w31:bool[])
    n316 = for {
      N: 6 -> [_]
      tunnel: "ABCDEF" -> [w593]
      tunnel: w31 -> [w586] mode=indexing
      shift-right: [w585] -> _
      shift-left: u16 0 ("length (rest)") -> [w591]
      shift-right: [w590] -> w25
      shift-left: cluster{string, u16}[] [] -> [w589]
      tunnel: w28 -> [w584]
      tunnel: w27 -> [w583]
      tunnel: [w584] -> w18
      tunnel: [w583] -> w26
      i -> [w592]
      # "Generate array of Device ID's, with sequential ID's"
      n317 = Equal?(x=w586, y=TRUE) -> (x = y?=w588:bool)
      n318 = case shown="True" w588 {
        tunnel: w593 -> [_ w604]
        tunnel: w592 -> [_ w603]
        tunnel: w591 -> [w594 w596]
        tunnel: [w595 w599] -> w590
        tunnel: w589 -> [w595 w597]
        tunnel: [w594 w600] -> w585
        frame False {
          # "ID was not included"
        }
        frame True {
          # "ID was included"
          n319 = String Subset(string=w604, offset (0)=w603, length (rest)=1 ("length (rest)")) -> (substring=w601:string)
          n320 = Bundle(w601, "length (rest)"=w596) -> (w598:cluster{string, "length (rest)":u16})  [unwired: 1 in]
          n321 = Increment(x=w596) -> (x+1=w600:u16)
          n322 = Build Array (concatenate)(w597, w598) -> (w599:cluster{string, "length (rest)":u16}[])
        }
      }
    }
    n323 = property on="Active Device" class="Ring (strict)"(error in=w18, "StringsAndValues[]"=w25) -> (error out=w17:errorcluster)  [unwired: 1 in, 1 out]
    n324 = for {
      tunnel: w26 -> [w581]
      tunnel: [w578] -> w22
      tunnel: w17 -> [w582]
      tunnel: [w577] -> w21
      tunnel: w25 -> [w579] mode=indexing
      tunnel: [w580] -> w24 mode=indexing
      tunnel: [w570] -> w23 mode=indexing
      tunnel: [w576] -> w20 mode=indexing
      tunnel: [nan ("Setpoint")] -> w19 mode=indexing
      tunnel: [w569] -> w16 mode=indexing
      # "Get measurement formats, unit ID's and the controller info"
      n325 = Unbundle(w579) -> (w570:string)  [unwired: 1 out]
      n326 = property on="Active Device" class="Ring (strict)" props=["Value"]() -> ()  [unwired: 2 in, 3 out]
      n327 = call "Read Measurement Format.vi"("Unit ID (A)"=w570, "error in"=w582, "VISA Session In"=w581) -> ("error out"=w573:errorcluster, "Data Frame Format"=w580:T10, "VISA Session Out"=w574:refnum<visa-resource-name>)  [unwired: 6 in]
      n328 = call "Read Software Version.vi"("Unit ID (A)"=w570, "error in"=w573, "VISA Session In"=w574) -> ("error out"=w572:errorcluster, "Software Version"=w569:u8, "VISA Session Out"=w571:refnum<visa-resource-name>)  [unwired: 6 in]
      n329 = call "Read Controller Info.vi"("Unit ID (A)"=w570, "error in"=w572, "Software Version"=w569, "VISA Session In"=w571) -> ("error out"=w577:errorcluster, "Controller Info out"=w576:T11, "VISA Session Out"=w578:refnum<visa-resource-name>)  [unwired: 4 in, 1 out]
    }
    n330 = while {
      shift-right: [w641] -> _
      shift-left: 0.0 ("Set Start Time (s)") -> [w644]
      shift-right: [w627] -> w40
      shift-left: w21 -> [w643]
      shift-right: [w608] -> w41
      shift-left: w22 -> [w642]
      tunnel: w23 -> [w606]
      shift-right: [w629] -> _
      shift-left: w24 -> [w636]
      shift-right: [w626] -> _
      shift-left: w20 -> [w624]
      shift-right: [w622] -> _
      shift-left: w19 -> [w621]
      shift-right: [w617] -> _
      shift-left: w16 -> [w617]
      tunnel: w12 -> [w615]
      stop <- w616 stop-if-true
      # "Acquire data for every device ID included at the requested data rate, then display only the selected device's data"
      n331 = call "Elapsed Time"("Set Start Time (s)"=w644) -> ("Get Start Time (s)"=w641:dbl, "Elapsed Time (s)"=w638:dbl)  [unwired: 11 in, 6 out]
      n332 = for {
        shift-right: [w673] -> w635
        shift-left: w643 -> [w676]
        shift-right: [w674] -> w634
        shift-left: w642 -> [w675]
        tunnel: w636 -> [w670] mode=indexing
        tunnel: w606 -> [w669] mode=indexing
        tunnel: [w668] -> w633 mode=indexing
        tunnel: [w667] -> w632 mode=indexing
        tunnel: [w666] -> w631 mode=indexing
        tunnel: [w665] -> w630 mode=indexing
        tunnel: [w664] -> w629 mode=indexing
        # "Acquire data for each device"
        n333 = call "Read Measurements.vi"("error in"=w676, "Data Frame Format In"=w670, "Unit ID (A)"=w669, "VISA Session In"=w675) -> ("error out"=w673:errorcluster, "Data Frame Format Out"=w664:T10, "Data Cluster"=w667:T3, "VISA Session Out"=w674:refnum<visa-resource-name>, "Unknown Dataframe Info"=w672:bool, "Error/Overrange/Unknown String"=w666:string, "Error Present"=w671:bool, "Range Exceeded"=w665:bool)
        n334 = Or(x=w672, y=w671) -> (x .or. y?=w668:bool)
      }
      n335 = local read "Z"() -> (w612:dbl[])
      n336 = Index Array(array=w612, index=1 ("index (row)")) -> (element=w610:dbl)
      "Active Device" <- w610
      n337 = To Long Integer(number=w610) -> (32bit integer=w619:i32)
      n338 = Multiply(x=1000.0 ("y"), y=w638) -> (x*y=→"Elapsed Time [ms]\n(all units)":dbl)
      n339 = Reciprocal(x=w638) -> ()  [unwired: 1 out]
      n340 = Wait (ms)(milliseconds to wait="Minimum time between \nreadings [ms] (all units)") -> ()  [unwired: 1 out]
      n341 = for {
        tunnel: w635 -> [w647]
        tunnel: [w646] -> w628
        tunnel: w634 -> [w648]
        tunnel: [w645] -> w607
        tunnel: w633 -> [w653] mode=indexing
        tunnel: w619 -> [w655]
        tunnel: w632 -> [w652] mode=indexing
        tunnel: w631 -> [w651] mode=indexing
        tunnel: w630 -> [w650] mode=indexing
        i -> [w654]
        # "Iterate over all sets of data, only display the one selected"
        n342 = Equal?(x=w655, y=w654) -> (x = y?=w649:bool)
        n343 = case shown="True" w649 {
          tunnel: w653 -> [_ w663]
          tunnel: w652 -> [_ w658]
          tunnel: w651 -> [_ w662]
          tunnel: w650 -> [_ w661]
          tunnel: w648 -> [w657 w659]
          tunnel: w647 -> [w656 w660]
          tunnel: [w656 w660] -> w646
          tunnel: [w657 w659] -> w645
          frame False {
            # "Do nothing"
          }
          frame True {
            # "Display data"
            "Range Exceeded" <- w661
            "Error Present" <- w663
            "Error Text" <- w662
            "Meas. Data (for active device)" <- w658
          }
        }
      }
      n344 = local read "Z"() -> (w614:dbl[])
      n345 = Index Array(array=w617, index=w619) -> (element=w618:u8)
      n346 = Index Array(array=w621, index=w619) -> (element=w609:dbl)
      n347 = Index Array(array=w614, index=0) -> (element=w605:dbl)
      n348 = Replace Array Subset(array=w621, new element=w605, index=w619) -> (w622:dbl[])
      n349 = Index Array(array=w606, index=w619) -> (element=w620:string)
      n350 = Index Array(array=w624, index=w619) -> (element=w623:T11)
      n351 = call "Write SetPoint_no prev.vi"("Setpoint"=w605, "Previous Setpoint"=w609, "Unit ID (A)"=w620, "error in"=w628, "Software Version"=w618, "Controller Info out"=w623, "VISA Session In"=w607) -> ("error out"=w627:errorcluster, "Controller Info out"=w625:T11, "VISA Session Out"=w608:refnum<visa-resource-name>)  [unwired: 1 in, 1 out]
      n352 = Replace Array Subset(array=w624, new element=w625, index=w619) -> (w626:T12)
      n353 = call <extravilib>:"Read.vi"("channel"=w615) -> ("element"=w616:bool)  [unwired: 1 in, 1 out]
    }
    n354 = while "Hold Setpoints" {
      tunnel: w12 -> [w53]
      stop <- w54 stop-if-true
      n355 = call-poly <vilib>:"Read Delimited Spreadsheet.vi"("file path (dialog if empty)"="Read File", "start of read offset (chars.:0)"=0, "delimiter (\\t)"="," ("delimiter (\\t)")) -> ("all rows"=w49:dbl[][])  [unwired: 7 in, 5 out]
      "all rows" <- w49
      n356 = Array Subset(array=w49, index (row)="Start From:") -> (w47:dbl[][])  [unwired: 3 in]
      "Setpoints" <- w47
      n357 = Array Size(array=w47) -> (size(s)=w56:i32[])
      n358 = Index Array(array=w56, index=0) -> (element=→"len_SP":i32)
      n359 = call <extravilib>:"Read.vi"("channel"=w53) -> ("element"=w54:bool)  [unwired: 1 in, 1 out]
    }
    n360 = VISA Close(VISA resource name=w41, error in (no error)=w40) -> (error out=w42:errorcluster)
    n361 = Initialize Array(0.0 ("element"), 2 ("dimension size")) -> (→"Z":dbl[])
    n362 = call <vilib>:"Simple Error Handler.vi"("error in (no error)"=w42) -> ("error?"=w4:bool)  [unwired: 4 in, 4 out]
    n363 = call "CalibrationAlerts.vi"("Alert Type (0)"=5, "Trigger"=w4) -> ()  [unwired: 10 in]
    n364 = call-poly <vilib>:"Write Delimited Spreadsheet.vi"("file path (dialog if empty)"="Write File", "1D data"=string[] ["Date/Time", "Time [hh:mm:ss]", "Device ID", "P_MFC [psia]", "T_MFC [C]", "Volume Flow [LPM]", "Mass Flow [SLPM]", "SP_MFC [LPM]", "T_SCh [C]", "Iter_#", "V_D [V]", "V_H [V]", "Iter_Duration [ms]", "C_SP_CH4 [ppm]", "C_SP_H2S [ppm]"], "append to file? (new file:F)"=TRUE, "delimiter (\\t)"="," ("delimiter (\\t)")) -> ()  [unwired: 10 in, 2 out]
    n365 = node-c288(w45) -> ()  [unwired: 1 out]
  }
